vi "PathPlanner_PathFinder_UpdateState.vi"(4 "eps_Little":dbl, 6 "Closed":set{T1}(c389), 7 "S":T1, 8 "G":map{i32, dbl}(c390), 9 "Incons":map{i32, T2}(c390), 10 "Open":map{i32, T2}(c390), 11 "RHS":map{i32, dbl}(c390)) -> (1 "Incons out":map{i32, T2}(c390), 2 "Open out":map{i32, T2}(c390), 3 "RHS out":map{i32, dbl}(c390))   [LabVIEW 2019]
uses:
  PathPlannerLib24/TypeDef/PathPlannerFinderGridPosition.ctl
  PathPlannerLib24/TypeDef/PathPlannerFinderDoublePair.ctl
  PathPlannerLib24/VI/PathPlanner_GridPosition_Get.vi
  PathPlannerLib24/VI/PathPlanner_GridPosition_New.vi
  PathPlannerLib24/VI/PathPlanner_PathFinder_Heuristic.vi
  PathPlannerLib24/VI/PathPlanner_PathFinder_IsCollision.vi
  PathPlannerLib24/VI/PathPlanner_GridPosition_Print.vi
  PathPlannerLib24/VI/PathPlanner_PathFinder_Globals.vi
  PathPlannerLib24/PathPlanner24.lvlib
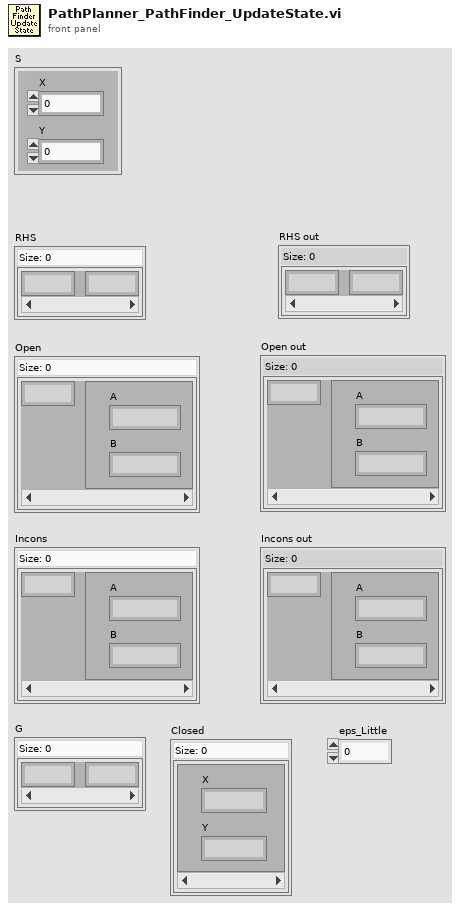
[diagram p1: front panel]
types:
  T1 = typedef "PathPlanner24.lvlib/PathPlannerFinderGridPosition.ctl" = cluster{"X":i32, "Y":i32}
  T2 = typedef "PathPlanner24.lvlib/PathPlannerFinderDoublePair.ctl" = cluster{"A":dbl, "B":dbl}
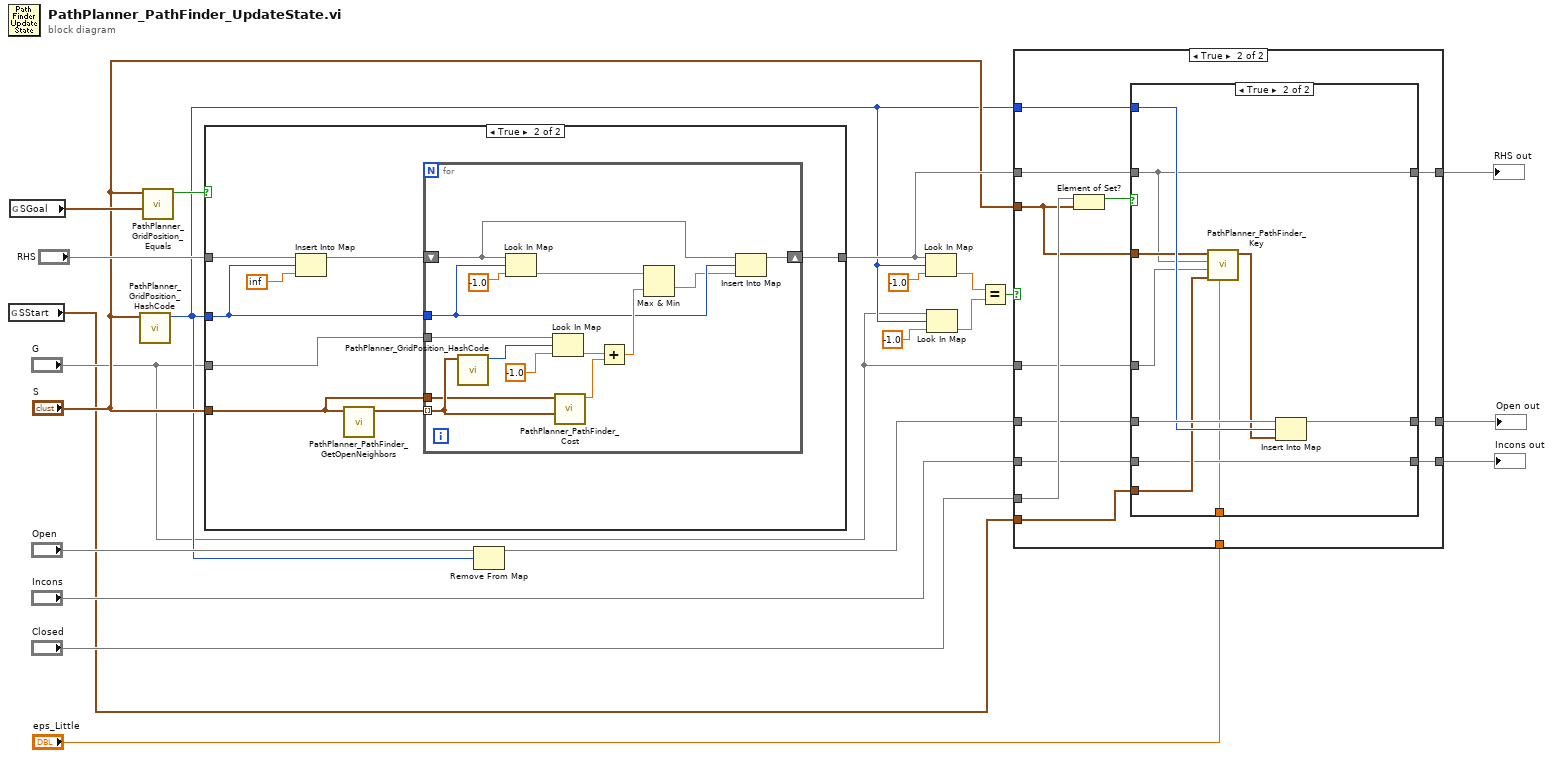
[diagram p0: block diagram]
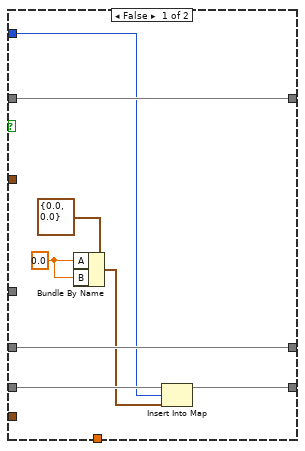
[diagram p3: hidden frame]
diagram:
  n1 = global read "PathPlanner_PathFinder_Globals.vi" "SStart"() -> (w2:T1)
  n2 = global read "PathPlanner_PathFinder_Globals.vi" "SGoal"() -> (w21:T1)
  n3 = call "PathPlanner_GridPosition_HashCode.vi"("GridPosition"="S") -> ("HashCode"=w4:i32)  [unwired: 10 in]
  n4 = call "PathPlanner_GridPosition_Equals.vi"("Other GridPosition"=w21, "GridPosition"="S") -> ("Equal"=w20:bool)  [unwired: 9 in]
  n5 = case shown="True" w20 {
    tunnel: "RHS" -> [w22 w30]
    tunnel: w4 -> [_ w26]
    tunnel: "S" -> [_ w24]
    tunnel: "G" -> [_ w25]
    tunnel: [w22 w23] -> w10
    frame False {
    }
    frame True {
      n6 = Insert Into Map(map in=w30, key=w26, value=inf) -> (map out=w27:map{i32, dbl})  [unwired: 2 out]
      n7 = call "PathPlanner_PathFinder_GetOpenNeighbors.vi"("GridPosition S"=w24) -> ("Open Neighbors"=w28:T1[])  [unwired: 10 in]
      n8 = for {
        tunnel: w28 -> [w37] mode=indexing
        shift-right: [w31] -> w23
        shift-left: w27 -> [w34]
        tunnel: w26 -> [w33]
        tunnel: w25 -> [w43]
        tunnel: w24 -> [w36]
        n9 = call "PathPlanner_GridPosition_HashCode.vi"("GridPosition"=w37) -> ("HashCode"=w42:i32)  [unwired: 10 in]
        n10 = Look In Map(map=w34, key=w33, default value=-1.0) -> (value=w40:dbl)  [unwired: 1 out]
        n11 = Look In Map(map=w43, key=w42, default value=-1.0) -> (value=w38:dbl)  [unwired: 1 out]
        n12 = call "PathPlanner_PathFinder_Cost.vi"("sGoalLoc"=w37, "sStartLoc"=w36) -> ("Cost"=w39:dbl)  [unwired: 9 in]
        n13 = Add(x=w38, y=w39) -> (x+y=w35:dbl)
        n14 = Max & Min(x=w40, y=w35) -> (min(x,y)=w32:dbl)  [unwired: 1 out]
        n15 = Insert Into Map(map in=w34, key=w33, value=w32) -> (map out=w31:map{i32, dbl})  [unwired: 2 out]
      }
    }
  }
  n16 = Remove From Map(10:w4, 11:"Open") -> (3:w13:map{i32, T2})  [unwired: 2 out]
  n17 = Look In Map(map=w10, key=w4, default value=-1.0) -> (value=w15:dbl)  [unwired: 1 out]
  n18 = Look In Map(map="G", key=w4, default value=-1.0) -> (value=w14:dbl)  [unwired: 1 out]
  n19 = Equal?(x=w15, y=w14) -> (x = y?=w11:bool)
  n20 = case shown="True" w11 {
    tunnel: w13 -> [w46 w58]
    tunnel: "Incons" -> [w45 w50]
    tunnel: w10 -> [w47 w55]
    tunnel: [w47 w51] -> w9
    tunnel: [w46 w52] -> w8
    tunnel: [w45 w49] -> w7
    tunnel: "Closed" -> [_ w60]
    tunnel: "S" -> [_ w56]
    tunnel: w4 -> [_ w57]
    tunnel: "G" -> [_ w54]
    tunnel: w2 -> [_ w53]
    tunnel: "eps_Little" -> [_ w48]
    frame False {
    }
    frame True {
      n21 = Element of Set?(10:w56, 11:w60) -> (3:w59:bool)
      n22 = case shown="True" w59 {
        tunnel: w58 -> [w65 w78]
        tunnel: w57 -> [w64 w77]
        tunnel: w56 -> [_ w76]
        tunnel: w55 -> [w66 w71]
        tunnel: w54 -> [_ w75]
        tunnel: w53 -> [_ w74]
        tunnel: [w65 w72] -> w52
        tunnel: [w66 w71] -> w51
        tunnel: w50 -> [w68 w70]
        tunnel: [w67 w70] -> w49
        tunnel: w48 -> [_ w69]
        frame False {
          w62 = 0.0 ("A")
          n23 = Bundle By Name(cluster=T2 {"A"=0.0, "B"=0.0} ("PathPlannerFinderDoublePair"), "A"=w62, "B"=w62) -> (w61:T2)
          n24 = Insert Into Map(map in=w68, key=w64, value=w61) -> (map out=w67:map{i32, T2})  [unwired: 2 out]
        }
        frame True {
          n25 = call "PathPlanner_PathFinder_Key.vi"("eps_little"=w69, "Sstart"=w74, "G"=w75, "RHS"=w71, "S"=w76) -> ("DoublePair"=w73:T2)  [unwired: 6 in]
          n26 = Insert Into Map(map in=w78, key=w77, value=w73) -> (map out=w72:map{i32, T2})  [unwired: 2 out]
        }
      }
    }
  }
  "RHS out" <- w9
  "Open out" <- w8
  "Incons out" <- w7
